vi "Initialization VI Name.vi"(11 "CD Template in":refnum<class "NIVS_Inline HW Interface (Inline-Async).lvclass">) -> (2 "Initialization VI Name":string)   [LabVIEW 2017, in "NIVS_Inline HW Interface (Inline-Async).lvclass"]
uses:
  NIVS_Inline HW Interface (Inline-Async).lvclass
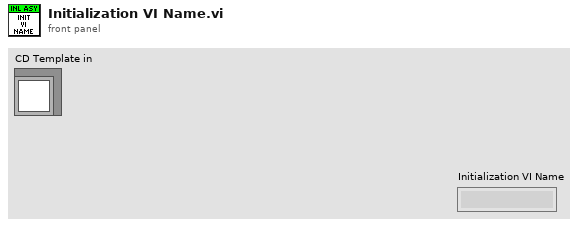
[diagram p1: front panel]
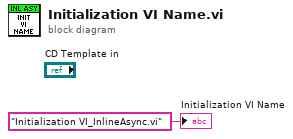
[diagram p0: block diagram]
diagram:
  "Initialization VI Name" <- "Initialization VI_InlineAsync.vi" ("Initialization VI Name")
